vi "plc read write.vi"(8 "error In":errorcluster, 9 "Length":i32=100, 10 "Start Address":i32=1350, 11 "connection ID IN":refnum<k5>) -> (0 "error out":errorcluster, 2 "Data":u32[](array[numeric]), 3 "connection ID OUT":refnum<k5>)   [LabVIEW 2015]
panel:
  out "substring 3":string
  out "substring 2":string
  out "bytes written1":i32
  # "ee"
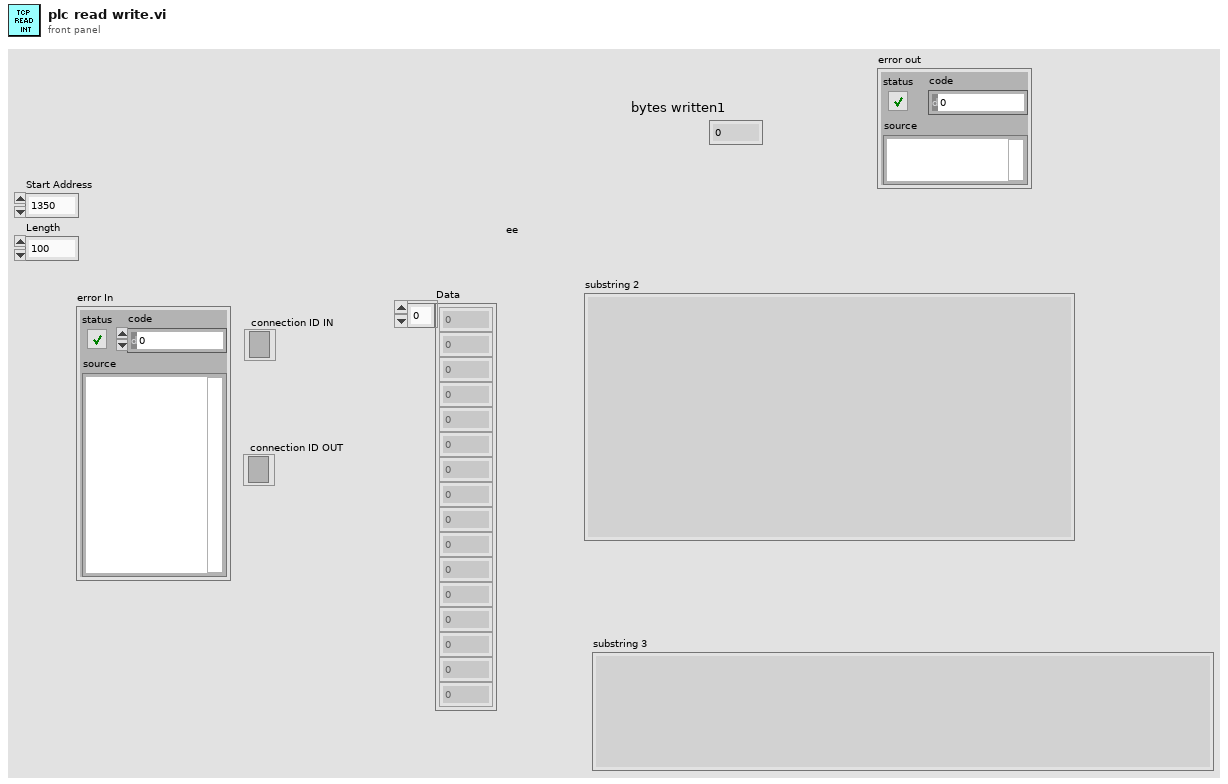
[diagram p1: front panel]
types:
  T1 = enum16{"Standard", "Buffered", "CRLF", "Immediate"}
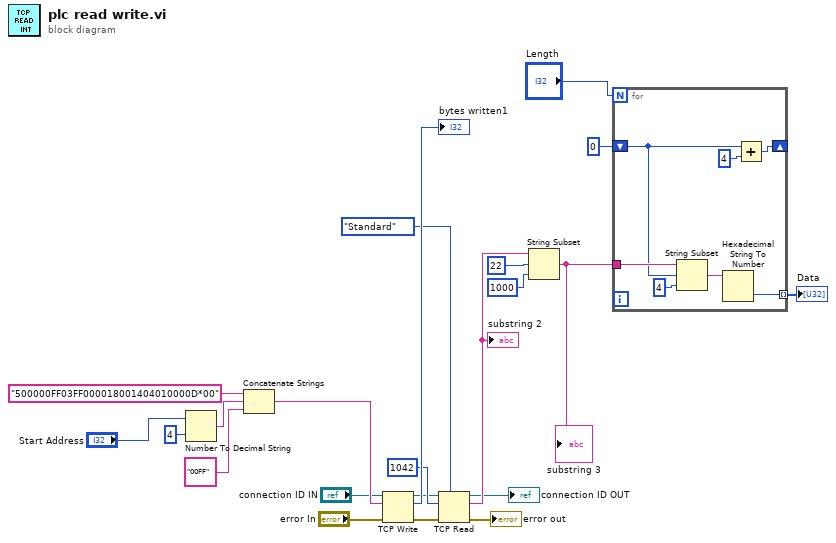
[diagram p0: block diagram]
diagram:
  n1 = Number To Decimal String(number="Start Address", width (-)=i16 4) -> (decimal integer string=w19:string)
  n2 = Concatenate Strings("500000FF03FF000018001404010000D*00", w19, "00FF" ("String")) -> (w21:string)
  n3 = TCP Write(connection ID="connection ID IN", data in=w21, error in (no error)="error In") -> (connection ID out=w14:refnum<k5>, bytes written=→"bytes written1":i32, error out=w12:errorcluster)  [unwired: 1 in]
  n4 = TCP Read(connection ID=w14, bytes to read=1042, error in (no error)=w12, 7:T1."Standard" ("mode (standard)")) -> (connection ID out=→"connection ID OUT":refnum<k5>, data out=w8:string, error out=→"error out":errorcluster)  [unwired: 1 in]
  "substring 2" <- w8
  n5 = String Subset(string=w8, offset (0)=22, length (rest)=1000 ("length (rest)")) -> (substring=w7:string)
  "substring 3" <- w7
  n6 = for {
    N: "Length" -> [_]
    shift-right: [w29] -> _
    shift-left: 0 -> [w26]
    tunnel: w7 -> [w27]
    tunnel: [w23] -> w6 mode=indexing
    n7 = String Subset(string=w27, offset (0)=w26, length (rest)=4 ("length (rest)")) -> (substring=w24:string)
    n8 = Hexadecimal String To Number(string=w24) -> (number=w23:u32)  [unwired: 2 in, 1 out]
    n9 = Add(x=w26, y=4) -> (x+y=w29:i32)
  }
  "Data" <- w6
